vi "Clean up.vi"(8 "error in (no error)":errorcluster, 11 "Analyze Timer in":refnum<class "Analyze Timer.lvclass">) -> (0 "error out":errorcluster, 3 "Analyze Timer out":refnum<class "Analyze Timer.lvclass">)   [LabVIEW 2009, in "Analyze.lvlib" / "Analyze Timer.lvclass"]
uses:
  Analyze Timer.lvclass
  Analyze BaseClass/Analyze BaseClass.lvclass
  Analyze Timer.lvclass/Analyze Timer.ctl
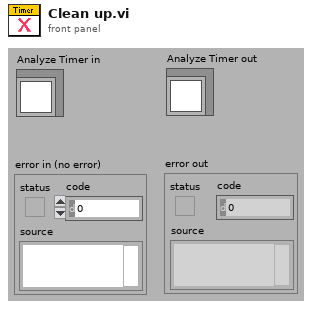
[diagram p1: front panel]
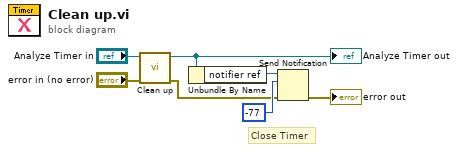
[diagram p0: block diagram]
diagram:
  # "Close Timer"
  n1 = call-parent "Clean up.vi"("error in (no error)"="error in (no error)", "Analyze BaseClass in"="Analyze Timer in") -> ("error out"=w2:errorcluster, "Analyze BaseClass out"=w4:refnum<class "Analyze Timer.lvclass">)  [unwired: 8 in]
  "Analyze Timer out" <- w4
  n2 = Unbundle By Name(w4) -> ("notifier ref"=w3:refnum<notifier>)
  n3 = Send Notification(notification=-77, notifier=w3, error in (no error)=w2) -> (error out=→"error out":errorcluster)  [unwired: 1 out]
